vi "Main - Find First Valid Result.vi"() -> ()   [LabVIEW 2011]
panel:
  out "# of iterations to find first valid sample set":i32
  out "# of Sample Sets":i32
  out "error out":errorcluster
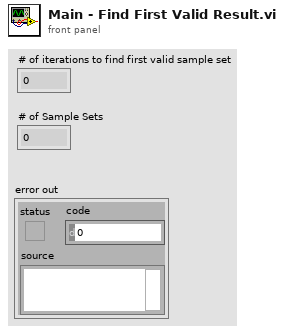
[diagram p1: front panel]
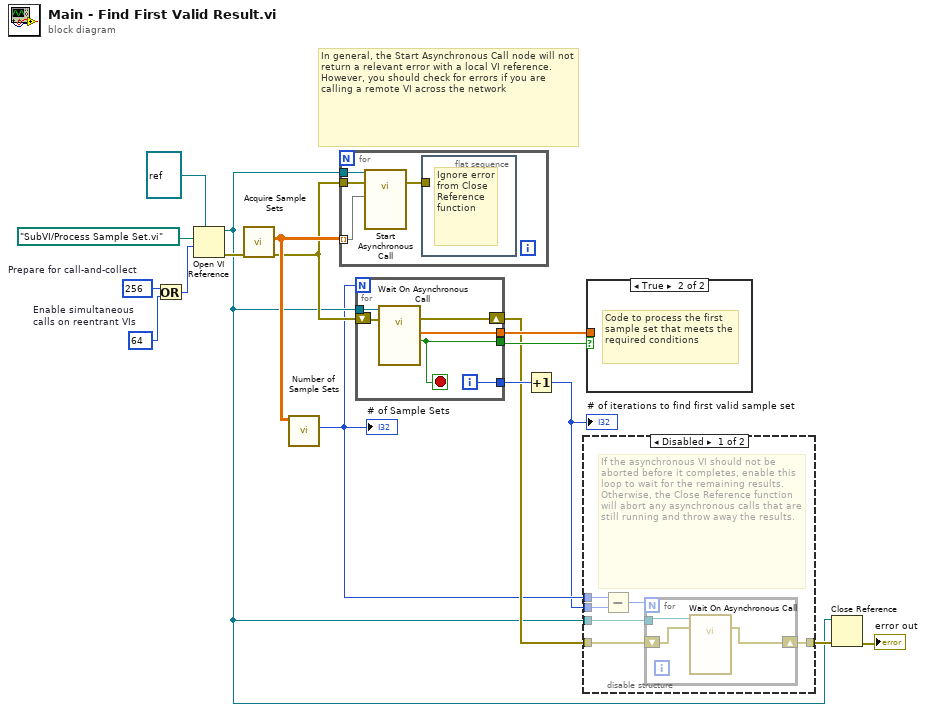
[diagram p0: block diagram]
diagram:
  w15 = 64  # Enable simultaneous calls on reentrant VIs
  w17 = 256  # Prepare for call-and-collect
  # "In general, the Start Asynchronous Call node will not return a relevant error with a local VI reference.\nHowever, you should check for errors if you are calling a remote VI across the network"
  n1 = Or(x=w17, y=w15) -> (x .or. y?=w16:i32)
  n2 = Open VI Reference(type specifier VI Refnum (for type only)=refnum<vi> refnum, vi path=path "SubVI/Process Sample Set.vi", options=w16) -> (vi reference=w3:refnum<vi>, error out=w12:errorcluster)  [unwired: 3 in]
  n3 = call "Acquire Sample Sets.vi"("error in (no error)"=w12) -> ("error out"=w5:errorcluster, "Sample Set"=w8:dbl[][])  [unwired: 9 in]
  n4 = call "Number of Sample Sets.vi"("Sample Set"=w8) -> ("Number of Sample Sets"=w2:i32)  [unwired: 10 in]
  "# of Sample Sets" <- w2
  n5 = for {
    tunnel: w8 -> [w20] mode=indexing
    tunnel: w3 -> [w21]
    tunnel: w5 -> [w19]
    n6 = call-by-ref "Start Asynchronous Call"(reference=w21, error in=w19, "Sample Set in"=w20) -> (error out=w18:errorcluster)  [unwired: 8 in, 4 out]
    n7 = flat-sequence {
      tunnel: w18 -> [_]
      frame #0 {
        # "Ignore error from Close Reference function"
      }
    }
  }
  n8 = for {
    N: w2 -> [_]
    tunnel: w3 -> [w27]
    tunnel: [w26] -> w9
    tunnel: [w25] -> w10
    tunnel: [w24] -> w11
    shift-right: [w22] -> w7
    shift-left: w5 -> [w23]
    i -> [w24]
    stop <- w25 stop-if-true
    n9 = call-by-ref "Wait On Asynchronous Call"(reference=w27, error in=w23) -> (error out=w22:errorcluster, "Valid?"=w25:bool, "Sample Set out"=w26:dbl[])  [unwired: 9 in, 2 out]
  }
  n10 = Increment(x=w11) -> (x+1=w1:i32)
  "# of iterations to find first valid sample set" <- w1
  n11 = disable-structure shown="Disabled" {
    disable-tunnel: w7 -> [w33 w37]
    disable-tunnel: [w32 w37] -> w6
    disable-tunnel: w3 -> [w31 _]
    disable-tunnel: w2 -> [w30 _]
    disable-tunnel: w1 -> [w29 _]
    frame Disabled {
      # "If the asynchronous VI should not be aborted before it completes, enable this loop to wait for the remaining results.\nOtherwise, the Close Reference function will abort any asynchronous calls that are still running and throw away the results."
      n12 = Subtract(x=w30, y=w29) -> (x-y=w28:i32)
      n13 = for {
        N: w28 -> [_]
        tunnel: w31 -> [w36]
        shift-right: [w34] -> w32
        shift-left: w33 -> [w35]
        n14 = call-by-ref "Wait On Asynchronous Call"(reference=w36, error in=w35) -> (error out=w34:errorcluster)  [unwired: 9 in, 4 out]
      }
    }
    frame Enabled {
    }
  }
  n15 = case shown="True" w10 {
    tunnel: w9 -> [_ _]
    frame False {
    }
    frame True {
      # "Code to process the first sample set that meets the required conditions"
    }
  }
  n16 = Close Reference(reference=w3, error in (no error)=w6) -> (error out=→"error out":errorcluster)
